vi "RB2 label the dot.vi"(1 "Dot Name":string="B", 2 "Dot Location":T2(array[cluster]), 3 "Num Dots":i32) -> (0 "Dot Data":T1)   [LabVIEW 2012]
doc: "This VI takes in dot location data, the type of dot as a string, and the number of dots. It outputs a cluster of the dot name, location in X, Y and the valid boolean."
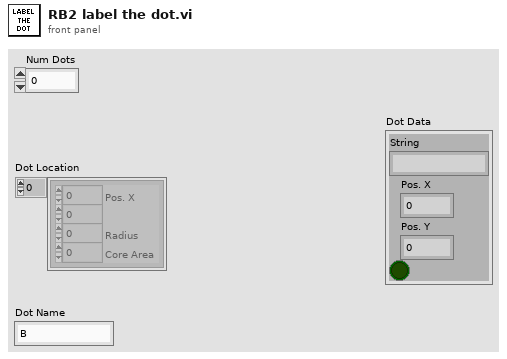
[diagram p1: front panel]
types:
  T1 = cluster{"String":string, "Pos. X":i32, "Pos. Y":i32, bool}
  T2 = cluster{"Pos. X":i32, "Pos. Y":i32, "Radius":i32, "Core Area":i32}[]
  T3 = cluster{"Pos. X":i32, "Pos. Y":i32, "Radius":i32, "Core Area":i32}
  T4 = cluster{"Dot Name":string, "Pos. X":i32, "Pos. Y":i32, bool}
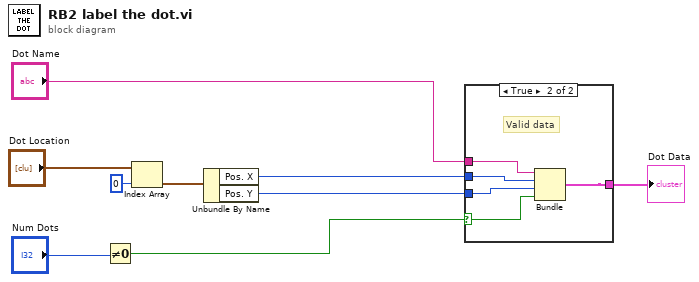
[diagram p0: block diagram]
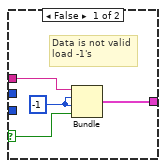
[diagram p2: hidden frame]
diagram:
  n1 = Not Equal To 0?(x="Num Dots") -> (x != 0?=w2:bool)
  n2 = Index Array(array="Dot Location", index=0) -> (element=w8:T3)
  n3 = Unbundle By Name(w8) -> ("Pos. X"=w6:i32, "Pos. Y"=w5:i32)
  n4 = case shown="True" w2 {
    selector: w2 -> [w12 w18]
    tunnel: [w10 w17] -> w4
    tunnel: w6 -> [_ w16]
    tunnel: w5 -> [_ w15]
    tunnel: "Dot Name" -> [w11 w14]
    frame False {
      w13 = i16 -1
      # "Data is not valid\nload -1's"
      n5 = Bundle("Dot Name"=w11, w13, w13, w12) -> (w10:cluster{"Dot Name":string, i16, i16, bool})  [unwired: 1 in]
    }
    frame True {
      # "Valid data"
      n6 = Bundle("Dot Name"=w14, "Pos. X"=w16, "Pos. Y"=w15, w18) -> (w17:T4)  [unwired: 1 in]
    }
  }
  "Dot Data" <- w4
